vi "Configure SMU Off-State.vi"(5 "Voltage Limit (20 V)":dbl=20.0, 6 "Source Off Function (1: Voltage)":i32(ring)=1 items=["Current", "Voltage"], 7 "Current Limit (0.001 A)":dbl=0.001, 8 "error in (no error)":errorcluster, 9 "Source Off Mode (0: Normal)":i32(ring) items=["Normal", "Zero", "High-Z"], 10 "Source Measure Unit Channel (0: Channel A)":i32(ring) items=["Channel A", "Channel B"], 11 "VISA resource name":refnum<visa-resource-name>) -> (0 "error out":errorcluster, 3 "VISA resource name out":refnum<visa-resource-name>)   [LabVIEW 2015, in "Keithley 2600 Series.lvlib"]
doc: "Configures the source function that is used when the output is turned off."
uses:
  Keithley 2600 Series.lvlib
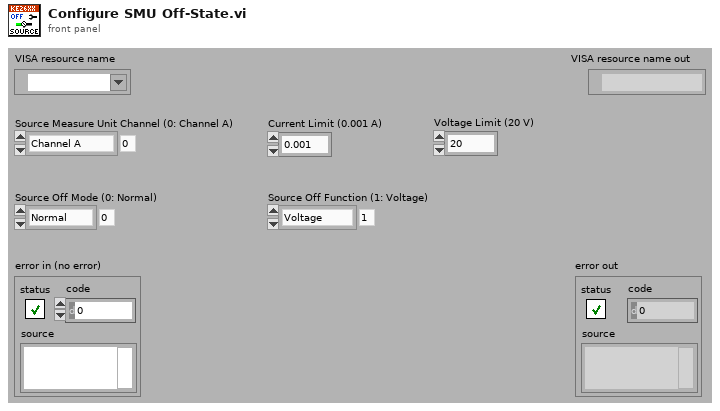
[diagram p1: front panel]
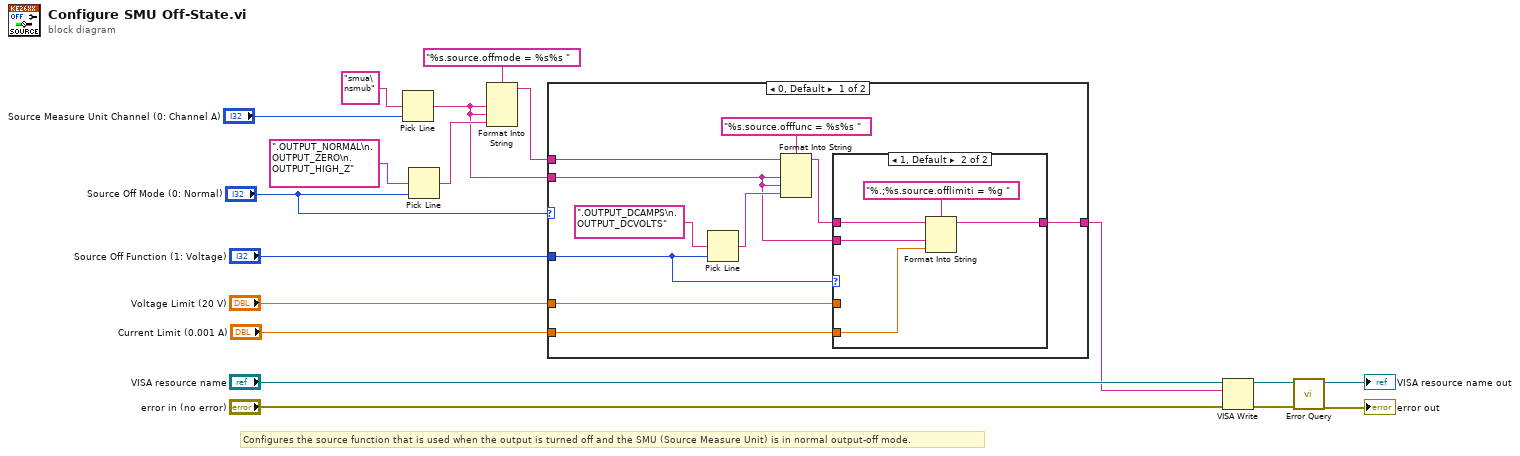
[diagram p0: block diagram]
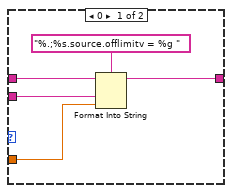
[diagram p2: hidden frame]
diagram:
  # "Configures the source function that is used when the output is turned off and the SMU (Source Measure Unit) is in normal output-off mode."
  n1 = Pick Line(multi-line string="smua\nsmub", line index="Source Measure Unit Channel (0: Channel A)") -> (output string=w4:string)  [unwired: 1 in]
  n2 = Pick Line(multi-line string=".OUTPUT_NORMAL\n.OUTPUT_ZERO\n.OUTPUT_HIGH_Z", line index="Source Off Mode (0: Normal)") -> (output string=w7:string)  [unwired: 1 in]
  n3 = Format Into String(format string="%s.source.offmode = %s%s ", w4, w4, w7) -> (resulting string=w3:string)  [unwired: 2 in, 1 out]
  n4 = case shown="0, Default" "Source Off Mode (0: Normal)" {
    tunnel: "Source Off Function (1: Voltage)" -> [w19 _]
    tunnel: "Voltage Limit (20 V)" -> [w24 _]
    tunnel: "Current Limit (0.001 A)" -> [w23 _]
    tunnel: w4 -> [w21 _]
    tunnel: w3 -> [w20 w39]
    tunnel: [w22 w39] -> w1
    frame 0, Default {
      n5 = Pick Line(multi-line string=".OUTPUT_DCAMPS\n.OUTPUT_DCVOLTS", line index=w19) -> (output string=w26:string)  [unwired: 1 in]
      n6 = Format Into String(format string="%s.source.offfunc = %s%s ", initial string=w20, w21, w21, w26) -> (resulting string=w25:string)  [unwired: 1 in, 1 out]
      n7 = case shown="1, Default" w19 {
        tunnel: w25 -> [w32 w37]
        tunnel: w24 -> [w31 _]
        tunnel: w23 -> [_ w36]
        tunnel: [w30 w35] -> w22
        tunnel: w21 -> [w29 w34]
        frame 0 {
          n8 = Format Into String(format string="%.;%s.source.offlimitv = %g ", initial string=w32, w29, w31) -> (resulting string=w30:string)  [unwired: 1 in, 1 out]
        }
        frame 1, Default {
          n9 = Format Into String(format string="%.;%s.source.offlimiti = %g ", initial string=w37, w34, w36) -> (resulting string=w35:string)  [unwired: 1 in, 1 out]
        }
      }
    }
    frame 1, 2 {
    }
  }
  n10 = VISA Write(VISA resource name="VISA resource name", write buffer=w1, error in (no error)="error in (no error)") -> (VISA resource name out=w16:refnum<visa-resource-name>, error out=w15:errorcluster)  [unwired: 1 out]
  n11 = call "Error Query.vi"("error in (no error)"=w15, "VISA resource name"=w16) -> ("error out"=→"error out":errorcluster, "VISA resource name out"=→"VISA resource name out":refnum<visa-resource-name>)  [unwired: 6 in, 2 out]
